vi "RIMAS Detector Conf.vi"(8 "Error In":errorcluster, 10 "Detector":u16, 11 "Detector Ref in":refnum<k5>) -> (0 "Error Out":errorcluster, 3 "Detector Ref out":refnum<k5>)   [LabVIEW 2024]
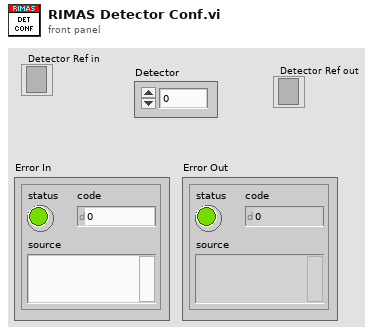
[diagram p1: front panel]
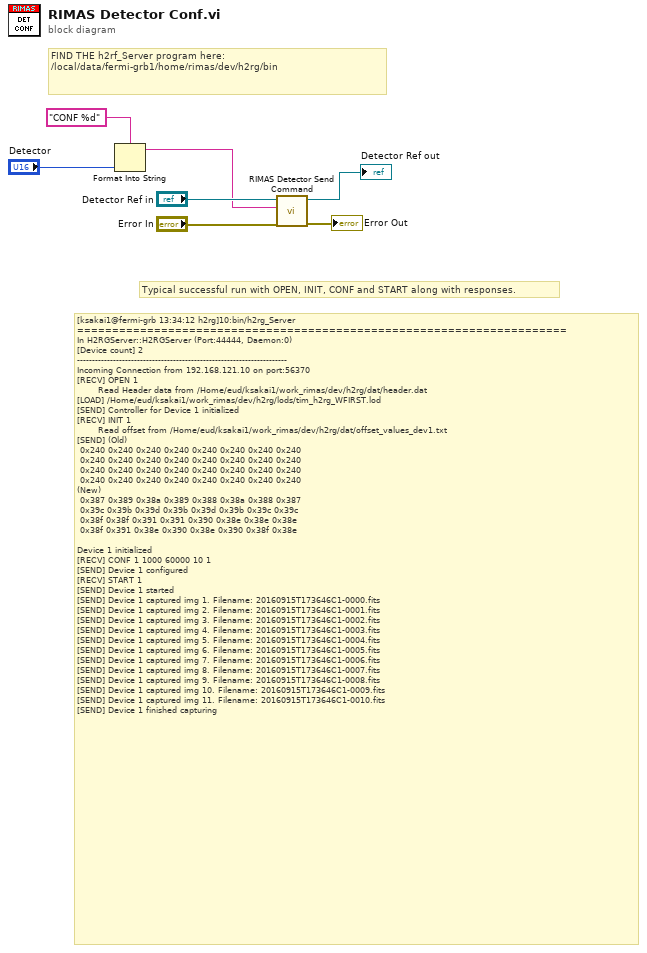
[diagram p0: block diagram]
diagram:
  # "FIND THE h2rf_Server program here:\n/local/data/fermi-grb1/home/rimas/dev/h2rg/bin"
  # "Typical successful run with OPEN, INIT, CONF and START along with responses."
  # "[ksakai1@fermi-grb 13:34:12 h2rg]10:bin/h2rg_Server\n======================================================================\nIn H2RGServer::H2RGServer (Port:44444, Daemon:0)\n[Device count] 2\n----------------------------------------------------------------------\nIncoming Connection from 192.168.121.10 on port:56370\n[RECV] OPEN 1\n       Read Header data from /Home/eud/ksakai1/work_rimas/dev/h2rg/dat/header.dat\n[LOAD] /Home/eud/ksakai1/work_rimas/dev/h2rg/lods/tim_h2rg_WFIRST.lod\n[SEND] Controller for Device 1 initialized\n[RECV] INIT 1\n       Read offset from /Home/eud/ksakai1/work_rimas/dev/h2rg/dat/offset_values_dev1.txt\n[SEND] (Old)\n 0x240 0x240 0x240 0x240 0x240 0x240 0x240 0x240\n 0x240 0x240 0x240 0x240 0x240 0x240 0x240 0x240\n 0x240 0x240 0x240 0x240 0x240 0x240 0x240 0x240\n 0x240 0x240 0x240 0x240 0x240 0x240 0x240 0x240\n(New)\n 0x387 0x389 0x38a 0x389 0x388 0x38a 0x388 0x387\n 0x39c 0x39b 0x39d 0x39b 0x39d 0x39b 0x39c 0x39c\n 0x38f 0x38f 0x391 0x391 0x390 0x38e 0x38e 0x38e\n 0x38f 0x391 0x38e 0x390 0x38e 0x390 0x38f 0x38e\n\nDevice 1 initialized\n[RECV] CONF 1 1000 60000 10 1\n[SEND] Device 1 configured\n[RECV] START 1\n[SEND] Device 1 started\n[SEND] Device 1 captured img 1. Filename: 20160915T173646C1-0000.fits\n[SEND] Device 1 captured img 2. Filename: 20160915T173646C1-0001.fits\n[SEND] Device 1 captured img 3. Filename: 20160915T173646C1-0002.fits\n[SEND] Device 1 captured img 4. Filename: 20160915T173646C1-0003.fits\n[SEND] Device 1 captured img 5. Filename: 20160915T173646C1-0004.fits\n[SEND] Device 1 captured img 6. Filename: 20160915T173646C1-0005.fits\n[SEND] Device 1 captured img 7. Filename: 20160915T173646C1-0006.fits\n[SEND] Device 1 captured img 8. Filename: 20160915T173646C1-0007.fits\n[SEND] Device 1 captured img 9. Filename: 20160915T173646C1-0008.fits\n[SEND] Device 1 captured img 10. Filename: 20160915T173646C1-0009.fits\n[SEND] Device 1 captured img 11. Filename: 20160915T173646C1-0010.fits\n[SEND] Device 1 finished capturing"
  n1 = Format Into String(format string="CONF %d", "Detector") -> (resulting string=w4:string)  [unwired: 2 in, 1 out]
  n2 = call "RIMAS Detector Send Command.vi"("Error In"="Error In", "Command"=w4, "Detector Ref"="Detector Ref in") -> ("Error Out"=→"Error Out":errorcluster, "Detector Ref dup"=→"Detector Ref out":refnum<k5>)  [unwired: 6 in, 1 out]
